vi "Weather Station UI.vi"(10 "Lower Limit":dbl=10.0, 11 "Upper Limit":dbl=30.0) -> (1 "Warning":string, 2 "Temperature History":dbl(graph))   [LabVIEW 2010]
doc: "This is the main VI in the Weather Station Project. It contains the user interface for a temperature warning system. \n\nUser inputs: Maximum Temperature, Minimum Temperature, Temperature Units.\nOutputs: Current Temperature, Warning State"
uses:
  Supporting Files/Weather Station States.ctl
panel:
  in  "Weather Data":dynamicdata(graph)
  in  "stop":bool
  in  "Wind Upper Limit":dbl(slide)=50.0 scale=0.0..100.0
  out "Wind Speed History":dbl(graph)
  # "Celsius"
  # "Temperature Ranges"
  # "Heat \nStroke"
  # "Freeze"
  # "kph"
  # "Maximum Safe Wind Speed"
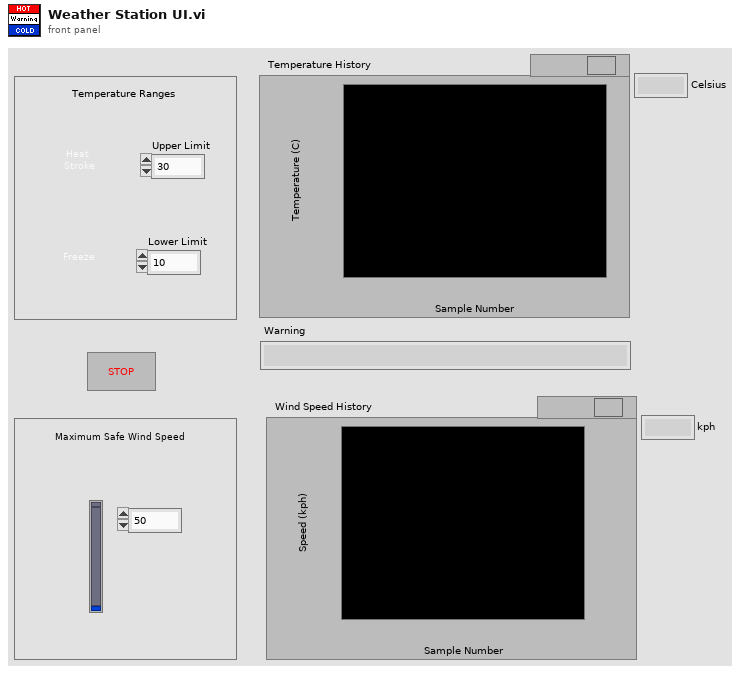
[diagram p1: front panel]
types:
  T1 = cluster{"Temperature":dbl, "T Upper Limit":dbl, "T Lower Limit":dbl, "Wind Speed":dbl, "Wind Upper Limit":dbl, "Warning":string, "Time":dbl}
  T2 = typedef "Weather Station States.ctl" = enum16{"Analysis", "Process UI", "Set Warning", "Data Log", "Stop"}
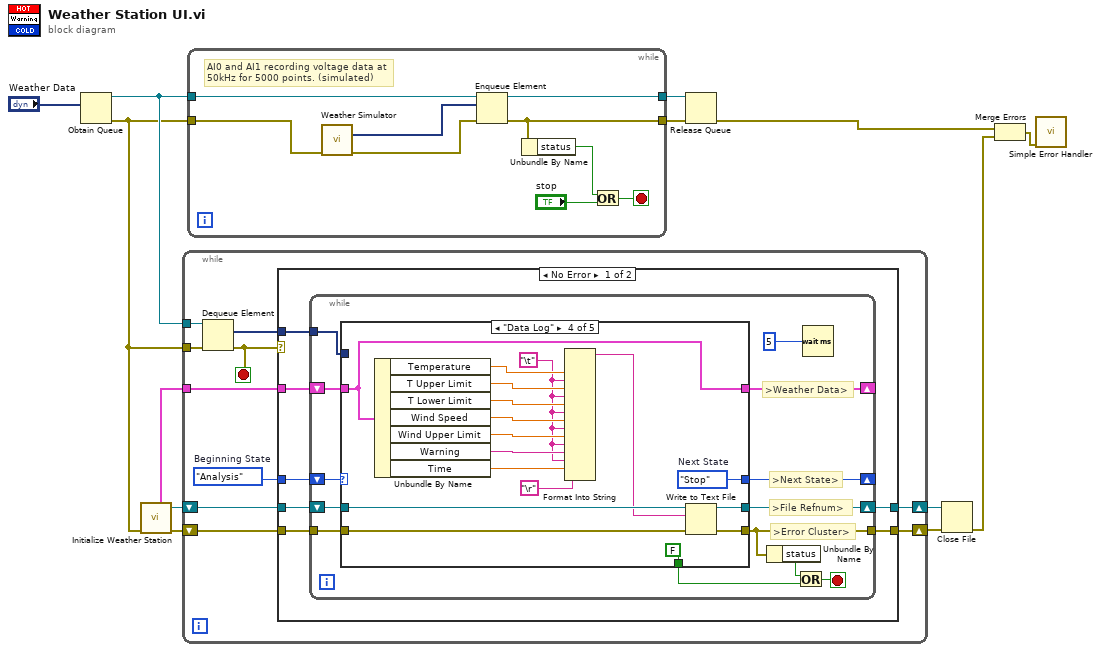
[diagram p0: block diagram]
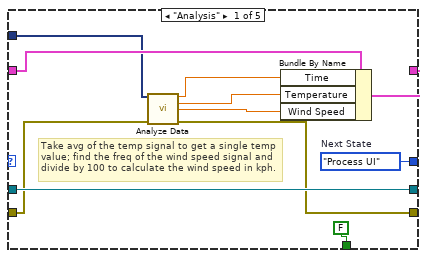
[diagram p2: hidden frame]
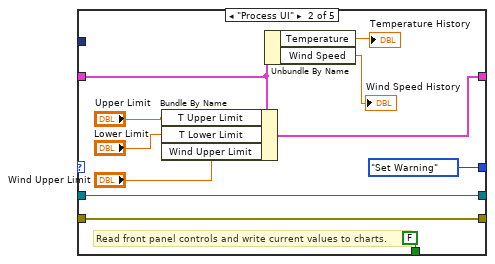
[diagram p3: hidden frame]
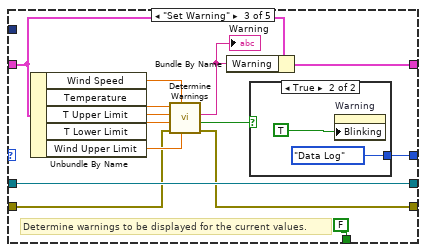
[diagram p4: hidden frame]
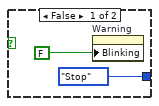
[diagram p5: hidden frame]
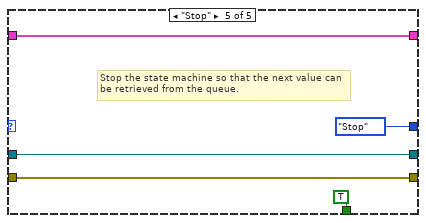
[diagram p6: hidden frame]
diagram:
  n1 = Obtain Queue(element data type="Weather Data") -> (queue out=w10:refnum<queue>, error out=w1:errorcluster)  [unwired: 3 in, 2 out]
  n2 = call "Initialize Weather Station.vi"("error in (no error)"=w1) -> ("error out"=w2:errorcluster, "file refnum"=w3:refnum<file>, "Weather Data"=w13:T1)  [unwired: 8 out]
  n3 = while {
    tunnel: w13 -> [w22]
    tunnel: w10 -> [w21]
    tunnel: w1 -> [w20]
    shift-right: [w23] -> w6
    shift-left: w3 -> [w19]
    shift-right: [w15] -> w5
    shift-left: w2 -> [w16]
    stop <- w18 stop-if-true
    w14 = Weather_Station_States."Analysis"  # Beginning State
    n4 = Dequeue Element(queue=w21, error in (no error)=w20) -> (element=w17:dynamicdata, error out=w18:errorcluster)  [unwired: 3 out]
    n5 = case shown="No Error" w18 {
      tunnel: [w30 w106] -> w23
      tunnel: w22 -> [w29 _]
      tunnel: w19 -> [w28 w106]
      tunnel: w17 -> [w27 _]
      tunnel: w16 -> [w25 w107]
      tunnel: [w26 w107] -> w15
      tunnel: w14 -> [w24 _]
      frame No Error {
        n6 = while {
          shift-right: [w43] -> _
          shift-left: w24 -> [w35]
          shift-right: [w32] -> w30
          shift-left: w28 -> [w42]
          shift-right: [w36] -> _
          shift-left: w29 -> [w39]
          tunnel: w27 -> [w34]
          tunnel: [w33] -> w26
          tunnel: w25 -> [w31]
          stop <- w41 stop-if-true
          # ">Error Cluster>"
          # ">Weather Data>"
          # ">File Refnum>"
          # ">Next State>"
          n7 = case shown="\"Data Log\"" w35 {
            tunnel: [w54 Weather_Station_States."Set Warning" ("Next State") w78 w100 Weather_Station_States."Stop" ("Next State")] -> w43
            tunnel: [w44 w56 w68 w97 w101] -> w33
            tunnel: w42 -> [w50 w55 w75 w96 w102]
            tunnel: [w51 w65 w76 w94 w103] -> w36
            tunnel: w39 -> [w52 w62 w77 w94 w103]
            tunnel: [FALSE ("stop") FALSE ("stop") FALSE ("stop") FALSE ("stop") TRUE ("stop")] -> w38
            tunnel: w34 -> [w49 _ _ _ _]
            tunnel: [w50 w55 w75 w98 w102] -> w32
            tunnel: w31 -> [w48 w56 w69 w84 w101]
            frame "Analysis" {
              w54 = Weather_Station_States."Process UI"  # Next State
              # "Take avg of the temp signal to get a single temp value; find the freq of the wind speed signal and divide by 100 to calculate the wind speed in kph."
              n8 = call "Analyze Data.vi"("Weather Data"=w49, "error in"=w48) -> ("Time"=w47:dbl, "Temperature"=w46:dbl, "Wind Speed"=w45:dbl, "error out"=w44:errorcluster)  [unwired: 2 in, 8 out]
              n9 = Bundle By Name(cluster=w52, "Time"=w47, "Temperature"=w46, "Wind Speed"=w45) -> (w51:T1)
            }
            frame "Process UI" {
              # "Read front panel controls and write current values to charts."
              n10 = Bundle By Name(cluster=w62, "T Upper Limit"="Upper Limit", "T Lower Limit"="Lower Limit", "Wind Upper Limit"="Wind Upper Limit") -> (w65:T1)
              n11 = Unbundle By Name(w62) -> ("Temperature"=→"Temperature History":dbl, "Wind Speed"=→"Wind Speed History":dbl)
            }
            frame "Set Warning" {
              # "Determine warnings to be displayed for the current values."
              n12 = Unbundle By Name(w77) -> ("Wind Speed"=w74:dbl, "Temperature"=w73:dbl, "T Upper Limit"=w72:dbl, "T Lower Limit"=w71:dbl, "Wind Upper Limit"=w70:dbl)
              n13 = call "Determine Warnings.vi"("Max Wind Speed"=w70, "Current Wind Speed"=w74, "error in (no error)"=w69, "Min Temp"=w71, "Max Temp"=w72, "Current Temp"=w73) -> ("error out"=w68:errorcluster, "Warning?"=w67:bool, "Warning Text"=w66:string)  [unwired: 3 out]
              "Warning" <- w66
              n14 = Bundle By Name(cluster=w77, "Warning"=w66) -> (w76:T1)
              n15 = case shown="True" w67 {
                tunnel: [Weather_Station_States."Stop" ("Next State") Weather_Station_States."Data Log" ("Next State")] -> w78
                frame False {
                  n16 = property on="Warning" class="Str"("Blinking"=FALSE) -> ()  [unwired: 2 in, 2 out]
                }
                frame True {
                  n17 = property on="Warning" class="Str"("Blinking"=TRUE) -> ()  [unwired: 2 in, 2 out]
                }
              }
            }
            frame "Data Log" {
              w86 = "\t"
              w100 = Weather_Station_States."Stop"  # Next State
              n18 = Unbundle By Name(w94) -> ("Temperature"=w93:dbl, "T Upper Limit"=w92:dbl, "T Lower Limit"=w91:dbl, "Wind Speed"=w90:dbl, "Wind Upper Limit"=w89:dbl, "Warning"=w88:string, "Time"=w87:dbl)
              n19 = Format Into String(w93, w86, w92, w86, w91, w86, w90, w86, w89, w86, w88, w86, w87, "\r") -> (resulting string=w95:string)  [unwired: 3 in, 1 out]
              n20 = Write to Text File(file (use dialog)=w96, text=w95, error in=w84) -> (refnum out=w98:refnum<file>, error out=w97:errorcluster)  [unwired: 2 out]
            }
            frame "Stop" {
              # "Stop the state machine so that the next value can be retrieved from the queue."
            }
          }
          n21 = Unbundle By Name(w33) -> ("status"=w40:bool)
          n22 = Or(x=w40, y=w38) -> (x .or. y?=w41:bool)
          n23 = Wait (ms)(milliseconds to wait=u32 5 ("y")) -> ()  [unwired: 1 out]
        }
      }
      frame Error {
      }
    }
  }
  n24 = while {
    tunnel: w10 -> [w116]
    tunnel: w1 -> [w110]
    tunnel: [w113] -> w12
    tunnel: [w115] -> w11
    stop <- w111 stop-if-true
    # "AI0 and AI1 recording voltage data at 50kHz for 5000 points. (simulated)"
    n25 = call "Weather Simulator.vi"("error in (no error)"=w110) -> ("Waveform Graph"=w108:dynamicdata, "error out"=w109:errorcluster)  [unwired: 13 out]
    n26 = Enqueue Element(queue=w116, element=w108, error in (no error)=w109) -> (queue out=w115:refnum<queue>, error out=w113:errorcluster)  [unwired: 2 out]
    n27 = Unbundle By Name(w113) -> ("status"=w112:bool)
    n28 = Or(x=w112, y="stop") -> (x .or. y?=w111:bool)
  }
  n29 = Release Queue(queue=w11, error in (no error)=w12) -> (error out=w8:errorcluster)  [unwired: 3 out]
  n30 = Close File(refnum=w6, error in=w5) -> (error out=w4:errorcluster)  [unwired: 1 out]
  n31 = Merge Errors(w8, w4) -> (w7:errorcluster)
  n32 = call <vilib>:"Simple Error Handler.vi"("error in (no error)"=w7) -> ()  [unwired: 1 in, 8 out]
